vi "Acquire.vi"(8 "error in (no error)":errorcluster, 10 "Msg in":T1, 11 "DG645 in":refnum<class "SMC100.lvclass">) -> (0 "error out":errorcluster, 1 "new command":string, 2 "Msg out":T1, 3 "DG645 out":refnum<class "SMC100.lvclass">)   [LabVIEW 2013, in "SMC100.lvclass"]
uses:
  SMC100.lvclass
  DriverMsg.ctl
  SMC100.lvclass/SMC100.ctl
  CompressAndUpdate(Numeric).vi
  source/Device Drivers/BaseDriver/BaseDriver.lvclass
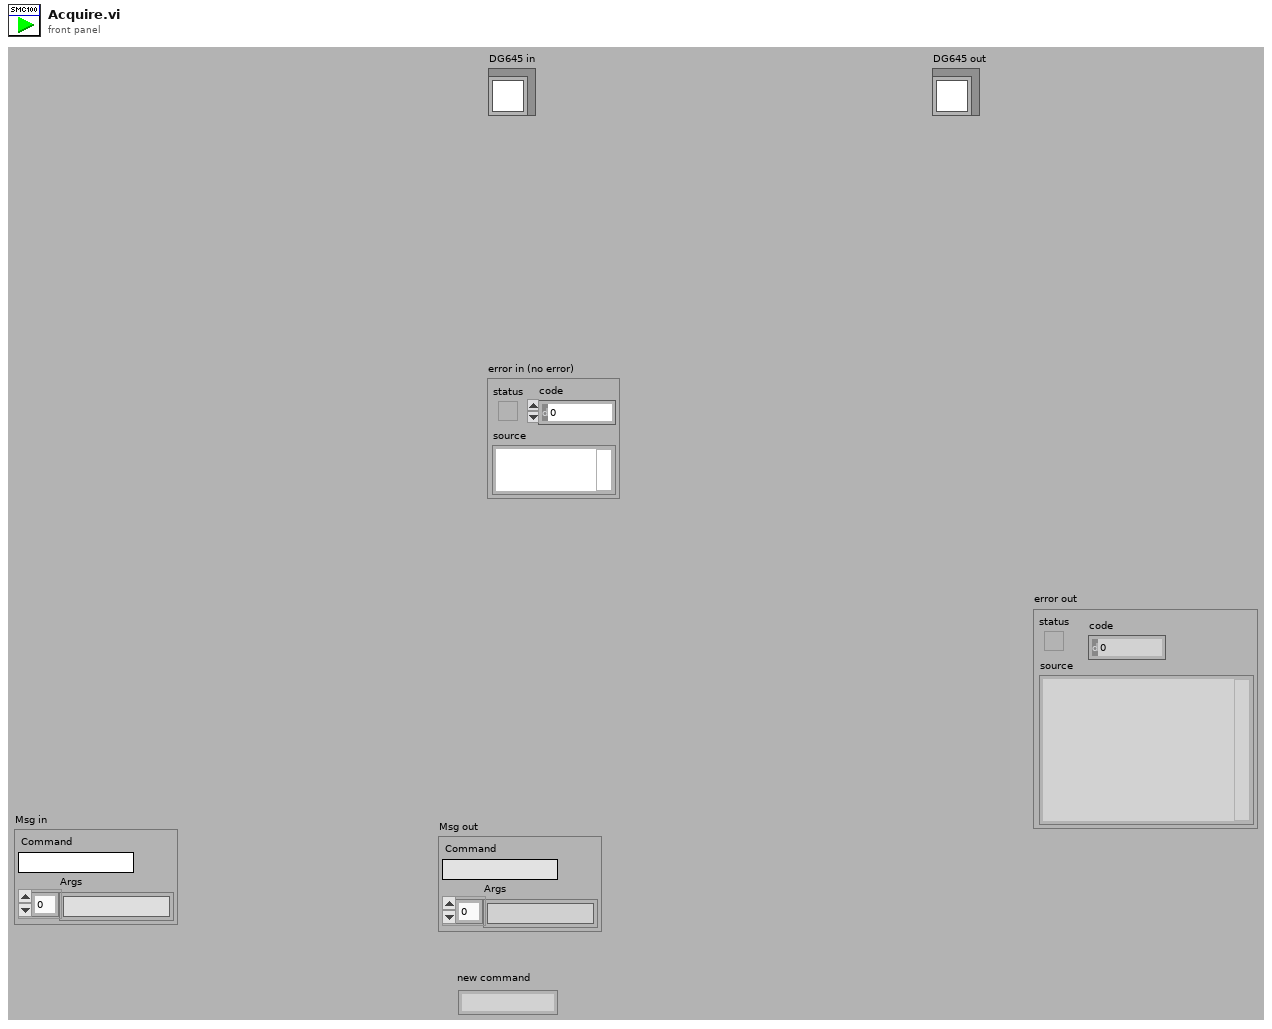
[diagram p1: front panel]
types:
  T1 = typedef "DriverMsg.ctl" = cluster{"Command":string, "Args":string[]}
  T2 = cluster{"VisaResourceName":string, "DeviceName":string, i32, "error out":errorcluster}
  T3 = cluster{"VISA resource name":refnum<visa-resource-name>, "Device name":string, "Controller address":i32, "error":errorcluster}
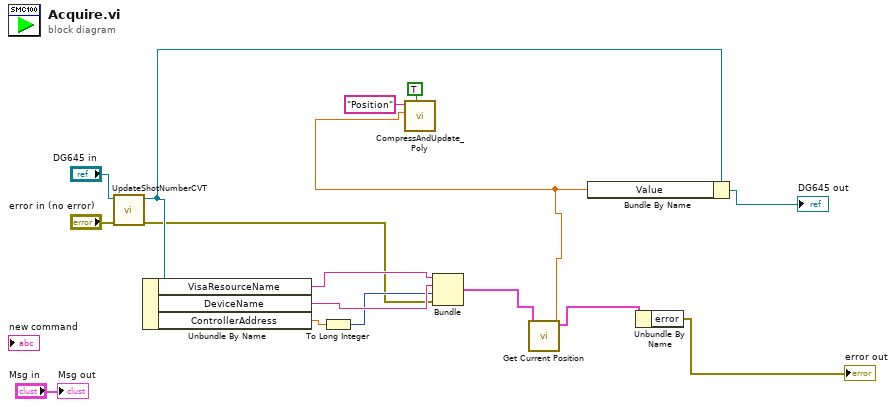
[diagram p0: block diagram]
diagram:
  n1 = call "UpdateShotNumberCVT.vi"("error in (no error)"="error in (no error)", "BaseDriver in"="DG645 in") -> ("error out"=w5:errorcluster, "BaseDriver out"=w10:refnum<class "SMC100.lvclass">)  [unwired: 8 in]
  n2 = Unbundle By Name(w10) -> ("VisaResourceName"=w8:string, "DeviceName"=w7:string, "ControllerAddress"=w9:dbl)
  n3 = To Long Integer(number=w9) -> (32bit integer=w6:i32)
  n4 = Bundle("VisaResourceName"=w8, "DeviceName"=w7, w6, "error out"=w5) -> (w3:T2)  [unwired: 1 in]
  n5 = call "Get Current Position.vi"("Connection Cluster in"=w3) -> ("Current position"=w1:dbl, "Connection Cluster out"=w2:T3)  [unwired: 8 in, 1 out]
  n6 = call-poly "CompressAndUpdate_Poly.vi"("force CVT update (false)"=TRUE, "Numeric"=w1, "command or variable name"="Position") -> ()  [unwired: 8 in, 1 out]
  n7 = Bundle By Name(cluster=w10, "Value"=w1) -> (→"DG645 out":refnum<class "SMC100.lvclass">)
  n8 = Unbundle By Name(w2) -> ("error"=→"error out":errorcluster)
  "Msg out" <- "Msg in"
